vi "subVI for splitting.vi"(8 "error in (no error)":errorcluster, 10 "queue":refnum<queue>, 11 "input string":string) -> (0 "error out":errorcluster, 2 "queue out":refnum<queue>, 3 "substring":string)   [LabVIEW 2012]
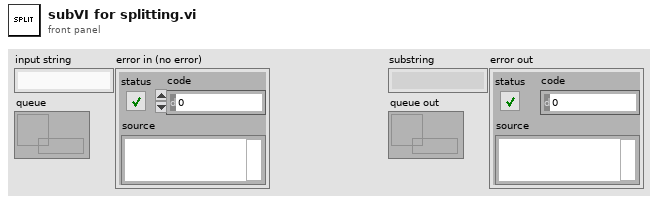
[diagram p1: front panel]
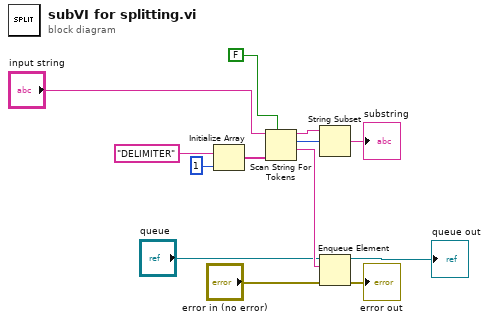
[diagram p0: block diagram]
diagram:
  n1 = Initialize Array("DELIMITER" ("element"), 1 ("dimension size")) -> (w12:string[])
  n2 = Scan String For Tokens(5:FALSE ("allow empty tokens? (F)"), 6:w12, 9:"input string") -> (1:w9:string, 2:w2:i32, 3:w13:string)  [unwired: 3 in, 1 out]
  n3 = String Subset(string=w13, offset (0)=w2) -> (substring=→"substring":string)  [unwired: 1 in]
  n4 = Enqueue Element(queue="queue", element=w9, error in (no error)="error in (no error)") -> (queue out=→"queue out":refnum<queue>, error out=→"error out":errorcluster)  [unwired: 1 in, 1 out]
